vi "PM100D_InitializeM1.vi"() -> (0 "error out":errorcluster, 1 "Instrument":string, 2 "VISA out":refnum<visa-resource-name>, 4 "SN":string)   [LabVIEW 2020]
doc: "This VI scans for connected devices, that can be selected in a dialog box. Next steps\n- setting timeout\n- performing identification query\n- configuring the operation register to '512'; flag gets to HI when a new measurement value is ready to fetch\n- clear operation register"
panel:
  in  "error in":errorcluster
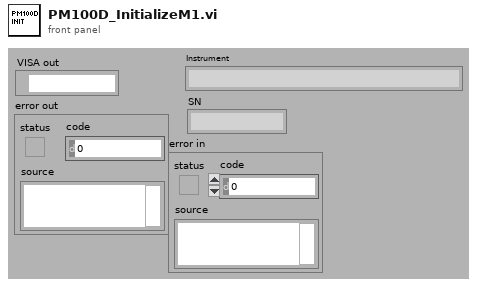
[diagram p1: front panel]
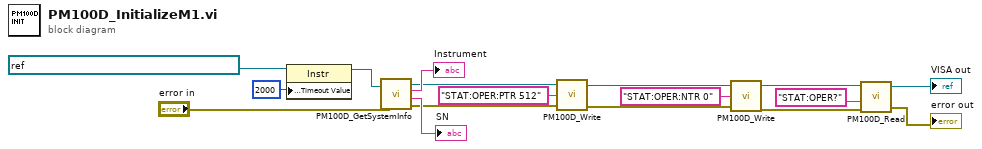
[diagram p0: block diagram]
diagram:
  n1 = property class="Instr"(reference=refnum<visa-resource-name> "USB0::0x1313::0x8078::P0045262::INSTR", "General Settings:Timeout Value"=u32 2000) -> (reference out=w14:refnum<visa-resource-name>)  [unwired: 1 in, 1 out]
  n2 = call "PM100D_GetSystemInfo.vi"("VISA in"=w14, "error in"="error in") -> ("VISA out"=w12:refnum<visa-resource-name>, "Instrument"=→"Instrument":string, "SN"=→"SN":string, "error out"=w10:errorcluster)
  n3 = call "PM100D_Write.vi"("error in (no error)"=w10, "Command"="STAT:OPER:PTR 512", "VISA in"=w12) -> ("error out"=w9:errorcluster, "VISA out"=w11:refnum<visa-resource-name>)
  n4 = call "PM100D_Write.vi"("error in (no error)"=w9, "Command"="STAT:OPER:NTR 0", "VISA in"=w11) -> ("error out"=w3:errorcluster, "VISA out"=w7:refnum<visa-resource-name>)
  n5 = call "PM100D_Read.vi"("error in (no error)"=w3, "Command"="STAT:OPER?", "VISA in"=w7) -> ("error out"=→"error out":errorcluster, "VISA out"=→"VISA out":refnum<visa-resource-name>)  [unwired: 1 in, 1 out]
